vi "Count Two Phase Encoder.vi"   [LabVIEW 2017, in "NI_Robotics_FPGA Utilities.lvlib"]
uses:
  <vilib>/robotics/Utilities/FPGA Utilities/NI_Robotics_FPGA Utilities.lvlib
  <vilib>/robotics/Utilities/NI_Robotics Utilities.lvlib
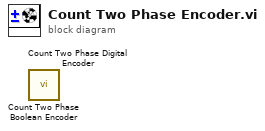
[diagram p0: block diagram]
diagram:
  n1 = call <vilib>:"Count Two Phase Boolean Encoder.vi"() -> ()  [unwired: 10 in, 2 out]
  n2 = call <vilib>:"Count Two Phase Digital Encoder.vi"() -> ()  [unwired: 10 in, 2 out]
